vi "XML - Get extra pages XML string.vi"(8 "error in (no error)":errorcluster, 11 "CD Wizard - Internal Data":T1) -> (0 "error out":errorcluster, 3 "Extra Pages XML string":string)   [LabVIEW 2015]
doc: "Creates the XML section for the extra pages. VeriStand needs for each extra page a section in the XML file to know the extra page and the corresponding configuration for the extra page."
uses:
  TypDef/CD Wizard - Internal data.ctl
  TypDef/CD Wizard - Execution Mode.ctl
  TypDef/CD Wizard - Extra Page Name and GUID.ctl
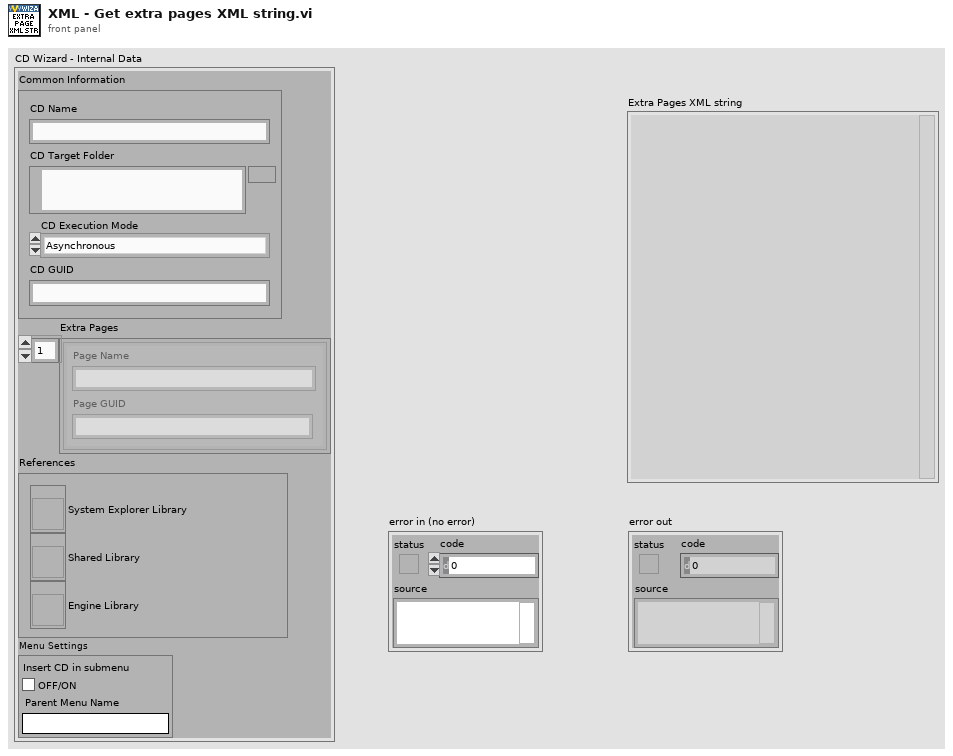
[diagram p1: front panel]
types:
  T1 = typedef "CD Wizard - Internal data.ctl" = cluster{"Common Information":cluster{"CD Name":string, "CD Target Folder":path, "CD Execution Mode":T2, "CD GUID":string}, "Extra Pages":T3[], "References":cluster{"System Explorer Library":refnum<vi>, "Shared Library":refnum<vi>, "Engine Library":refnum<vi>}, "Menu Settings":cluster{"Insert CD in submenu":bool, "Parent Menu Name":string}}
  T2 = typedef "CD Wizard - Execution Mode.ctl" = enum16{"Asynchronous", "Inline HW Interface", "Inline Model Interface", "Inline Timing and Sync", "Asynchronous Timing and Sync"}
  T3 = typedef "CD Wizard - Extra Page Name and GUID.ctl" = cluster{"Page Name":string, "Page GUID":string}
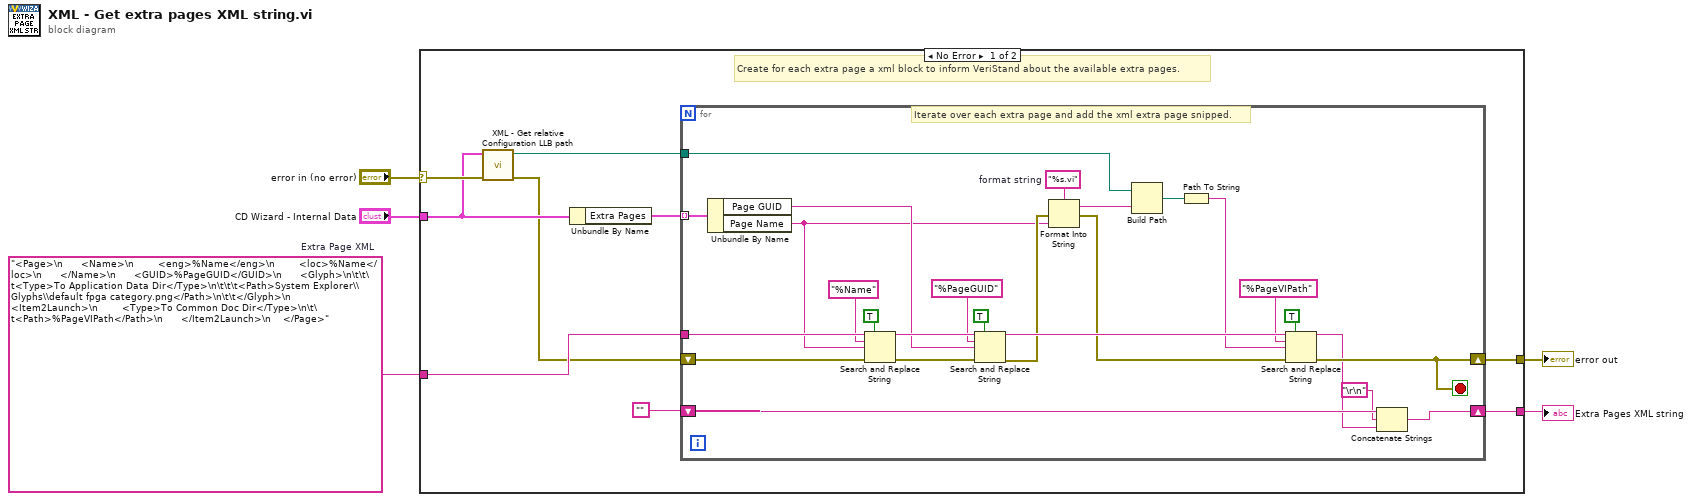
[diagram p0: block diagram]
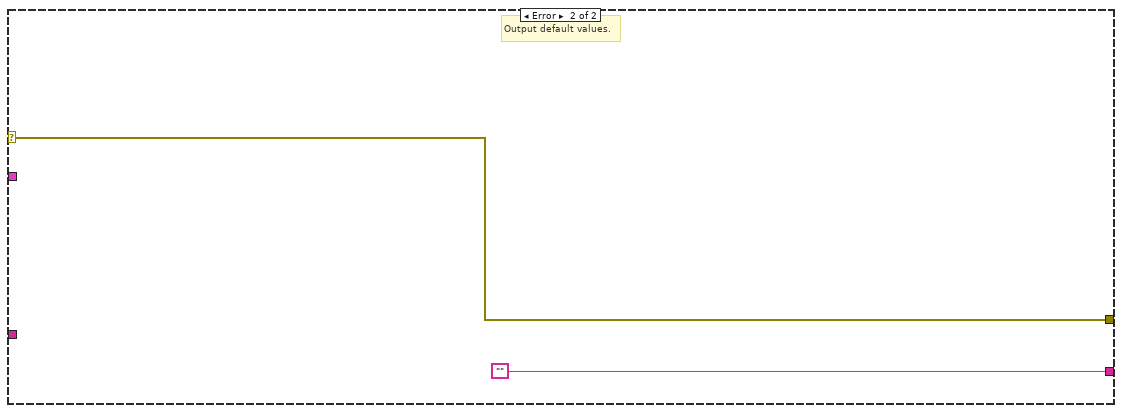
[diagram p2: hidden frame]
diagram:
  w2 = "<Page>\n      <Name>\n        <eng>%Name</eng>\n        <loc>%Name</loc>\n      </Name>\n      <GUID>%PageGUID</GUID>\n      <Glyph>\n\t\t\t<Type>To Application Data Dir</Type>\n\t\t\t<Path>System Explorer\\Glyphs\\default fpga category.png</Path>\n\t\t</Glyph>\n      <Item2Launch>\n        <Type>To Common Doc Dir</Type>\n\t\t<Path>%PageVIPath</Path>\n      </Item2Launch>\n    </Page>"  # Extra Page XML
  n1 = case shown="No Error" "error in (no error)" {
    selector: "error in (no error)" -> [w11 w42]
    tunnel: [w7 w42] -> w4
    tunnel: "CD Wizard - Internal Data" -> [w10 _]
    tunnel: w2 -> [w12 _]
    tunnel: [w8 ""] -> w1
    frame No Error {
      # "Create for each extra page a xml block to inform VeriStand about the available extra pages."
      n2 = call "XML - Get relative Configuration LLB path.vi"("error in (no error)"=w11, "CD Wizard - Internal Data"=w10) -> ("error out"=w9:errorcluster, "Relative Configuration LLB path"=w6:path)  [unwired: 8 in]
      n3 = Unbundle By Name(w10) -> ("Extra Pages"=w13:T3[])
      n4 = for {
        tunnel: w12 -> [w40]
        shift-right: [w31] -> w8
        shift-left: "" -> [w30]
        tunnel: w13 -> [w29] mode=indexing
        shift-right: [w25] -> w7
        shift-left: w9 -> [w26]
        tunnel: w6 -> [w18]
        stop <- w25 stop-if-true
        w24 = "%s.vi"  # format string
        # "Iterate over each extra page and add the xml extra page snipped."
        n5 = Unbundle By Name(w29) -> ("Page GUID"=w27:string, "Page Name"=w21:string)
        n6 = Search and Replace String(replace all?=TRUE ("replace all? (F)"), input string=w40, search string="%Name", replace string=w21, error in=w26) -> (result string=w36:string, error out=w28:errorcluster)  [unwired: 5 out]
        n7 = Search and Replace String(replace all?=TRUE ("replace all? (F)"), input string=w36, search string="%PageGUID", replace string=w27, error in=w28) -> (result string=w33:string, error out=w22:errorcluster)  [unwired: 5 out]
        n8 = Format Into String(format string=w24, error in=w22, w21) -> (resulting string=w17:string, error out=w23:errorcluster)  [unwired: 1 in]
        n9 = Build Path(base path=w18, name or relative path=w17) -> (appended path=w20:path)
        n10 = Path To String(path=w20) -> (string=w19:string)
        n11 = Search and Replace String(replace all?=TRUE ("replace all? (F)"), input string=w33, search string="%PageVIPath", replace string=w19, error in=w23) -> (result string=w15:string, error out=w25:errorcluster)  [unwired: 5 out]
        n12 = Concatenate Strings(w30, "\r\n", w15) -> (w31:string)
      }
    }
    frame Error {
      # "Output default values."
    }
  }
  "error out" <- w4
  "Extra Pages XML string" <- w1
